vi "FW_GetImageName.vi"(8 "error in":errorcluster, 11 "Image":T1) -> (0 "error out":errorcluster, 3 "before match":string)   [LabVIEW 2021, in "Framework_lib.lvlib"]
uses:
  QMH/Framework_lib.lvlib
  <vilib>/vision/Image Controls.llb/IMAQ Image.ctl
  <vilib>/regexp/Match Regular Expression.xnode
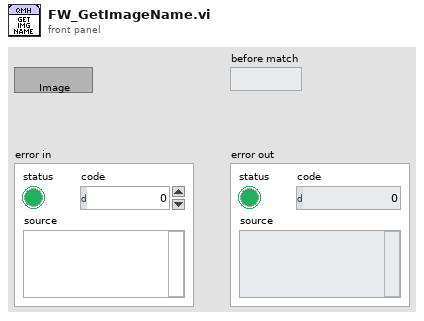
[diagram p1: front panel]
types:
  T1 = typedef "IMAQ Image.ctl" = refnum<image>
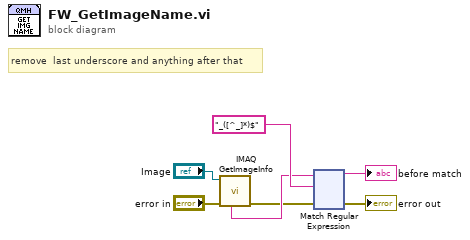
[diagram p0: block diagram]
diagram:
  # "remove  last underscore and anything after that"
  n1 = call "IMAQ GetImageInfo"("error in (no error)"="error in", "Image"="Image") -> ("error out"=w1:errorcluster, "Image Name"=w6:string)  [unwired: 2 in, 6 out]
  n2 = xnode "Match Regular Expression"("input string"=w6, "regular expression"="_([^_]*)$", "error in"=w1) -> ("before match"=→"before match":string, "error out"=→"error out":errorcluster)  [unwired: 3 in, 3 out]
